vi "Draw.vi"(7 "Stimulus Snippet":T1, 8 "error in (no error)":errorcluster, 9 "StimulusImageIn":T2, 10 "CalibrationImage":T2, 11 "TriggerOnTurnsTwoColors in":refnum<class "TriggerOnTurnsTwoColors.lvclass">) -> (0 "error out":errorcluster, 1 "StimulusImageOut":T2, 3 "TriggerOnTurnsTwoColors out":refnum<class "TriggerOnTurnsTwoColors.lvclass">)   [LabVIEW 2019, in "TriggerOnTurnsTwoColors.lvclass"]
uses:
  TriggerOnTurnsTwoColors.lvclass
  <vilib>/vision/Image Controls.llb/IMAQ Image.ctl
  StimulusSnippetCluster.ctl
  TriggerOnTurnsTwoColors.lvclass/TriggerOnTurnsTwoColors.ctl
  ParametersGlobal.vi
  <vilib>/vision/NI_Vision_Development_Module.lvlib
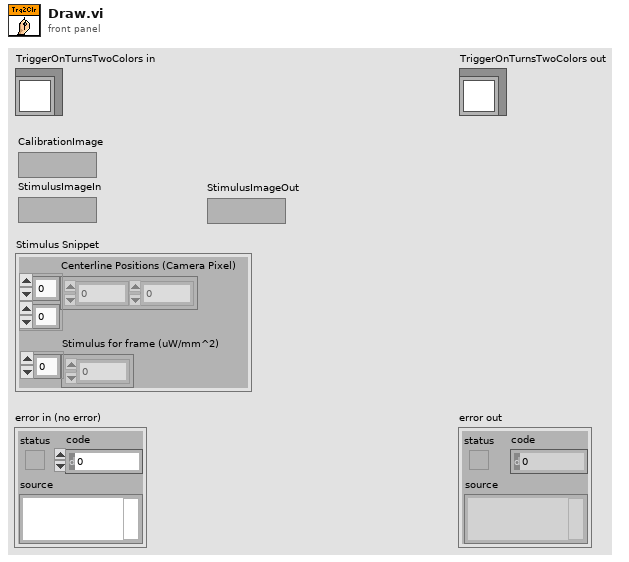
[diagram p1: front panel]
types:
  T1 = typedef "StimulusSnippetCluster.ctl" = cluster{"Centerline Positions (Camera Pixel)":sgl[][], "Stimulus for frame (uW/mm^2)":sgl[]}
  T2 = typedef "IMAQ Image.ctl" = refnum<image>
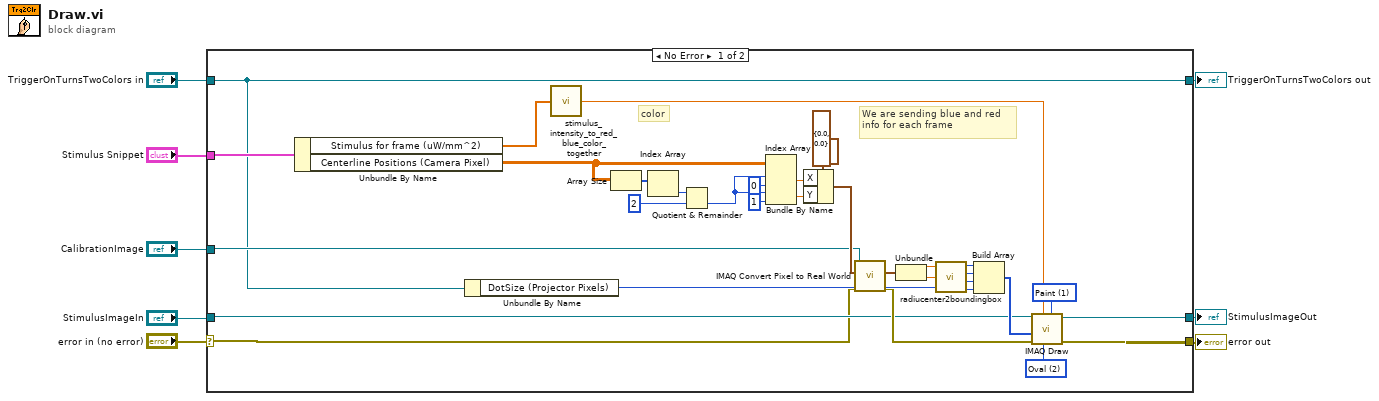
[diagram p0: block diagram]
diagram:
  n1 = case shown="No Error" "error in (no error)" {
    selector: "error in (no error)" -> [w15 w43]
    tunnel: [w13 w43] -> w5
    tunnel: [w12 w42] -> w1
    tunnel: "TriggerOnTurnsTwoColors in" -> [w12 w42]
    tunnel: [w14 w41] -> w6
    tunnel: "StimulusImageIn" -> [w16 w41]
    tunnel: "Stimulus Snippet" -> [w18 _]
    tunnel: "CalibrationImage" -> [w17 _]
    frame No Error {
      w24 = u16 1 items=["Frame", "Paint", "Invert Frame", "Invert Paint"] ("Draw Mode")
      w23 = u16 2 items=["Line", "Rectangle", "Oval"] ("Shape to draw")
      # "We are sending blue and red info for each frame"
      # "color"
      n2 = Unbundle By Name(w18) -> ("Stimulus for frame (uW/mm^2)"=w10:sgl[], "Centerline Positions (Camera Pixel)"=w11:sgl[][])
      n3 = Unbundle By Name(w12) -> ("DotSize (Projector Pixels)"=w36:i32)
      n4 = call "stimulus_intensity_to_red_blue_color_together.vi"("StimulusIntensityForFrame"=w10) -> ("StimulusColorForFrame"=w9:sgl)
      n5 = Array Size(array=w11) -> (size(s)=w38:i32[])
      n6 = Index Array(array=w38) -> (element=w39:i32)  [unwired: 1 in]
      n7 = Quotient & Remainder(x=w39, y=2) -> (floor(x/y)=w40:i32)  [unwired: 1 out]
      n8 = Index Array(array=w11, index (row) #1=w40, index (col) #1=0 ("disabled index (col)"), index (row) #2=w40, index (col) #2=1 ("disabled index (col)")) -> (element #1=w34:sgl, element #2=w35:sgl)
      n9 = Bundle By Name(cluster=cluster{"X":sgl, "Y":sgl} {"X"=0.0, "Y"=0.0} ("Camera Point"), "X"=w34, "Y"=w35) -> (w37:cluster{"X":sgl, "Y":sgl})
      n10 = call "IMAQ Convert Pixel to Real World"("error in (no error)"=w15, "Pixel Coordinates"=w37, "Calibrated Image"=w17) -> ("error out"=w33:errorcluster, "Real World Coordinates"=w32:cluster{"X":sgl, "Y":sgl})  [unwired: 3 in, 4 out]
      n11 = Unbundle(w32) -> ("X"=w30:sgl, "Y"=w31:sgl)
      n12 = call "radiucenter2boundingbox.vi"("Radius"=w36, "ycenter"=w31, "xcenter"=w30) -> ("Bottom"=w29:i32, "Right"=w28:i32, "Top"=w27:i32, "Left"=w26:i32)  [unwired: 2 in]
      n13 = Build Array(w26, w27, w28, w29) -> (w25:i32[])
      n14 = call "IMAQ Draw"("Draw Mode"=w24, "Shape to draw"=w23, "Pixel Color"=w9, "error in (no error)"=w33, "Coordinates"=w25, "Image Src"=w16) -> ("error out"=w13:errorcluster, "Image Dst Out"=w14:T2)  [unwired: 4 in]
    }
    frame Error {
    }
  }
  "error out" <- w5
  "TriggerOnTurnsTwoColors out" <- w1
  "StimulusImageOut" <- w6
